vi "Passing Arrays as Read-Only ndarrays.vi"() -> ()   [LabVIEW 2020]
uses:
  6d5f1638-640c-4e20-b011-0cee3ae60b95.vi
  688a6956-cd2d-4b8a-a8be-e172edc5432f.vi
  G-Embedded-Python-Interpreter-Toolkit/Null Py Object Refnum.vi
  6d5f1638-640c-4e20-b011-0cee3ae60b95.vi/96ddca92-7bbf-40e2-a1a5-d32f291eb6af.vi
  688a6956-cd2d-4b8a-a8be-e172edc5432f.vi/6c7a13f1-33d3-431d-8188-904cac5422b3.vi
  G-Embedded-Python-Interpreter-Toolkit/Python Object Reference to Pointer Sized Ref.vi
  G-Embedded-Python-Interpreter-Toolkit/Pointer Sized Ref to Python Object Reference.vi
  G-Embedded-Python-Interpreter-Toolkit/Merge Call Library Errors.vi
  G-Embedded-Python-Interpreter-Toolkit/G-Embedded-Python-Interpreter-Toolkit.lvlib
panel:
  out "Average History":dbl(graph)
  out "Sample History":dbl[](graph)
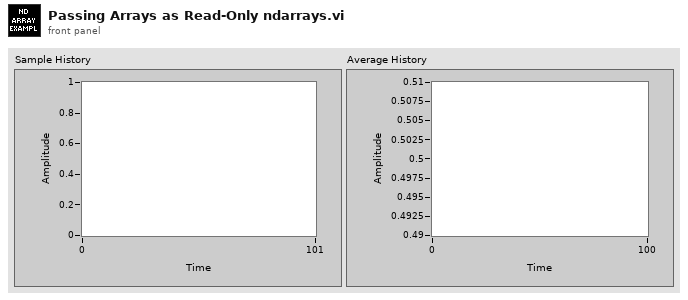
[diagram p1: front panel]
types:
  T1 = typedef "G-Embedded-Python-Interpreter-Toolkit.lvlib/Python Object Reference.ctl" = refnum<k1>
  T2 = typedef "G-Embedded-Python-Interpreter-Toolkit.lvlib/Type Information.ctl" = cluster{"Type":T3, "Array Dimensions":u8}
  T3 = typedef "NI_Data Type.lvlib/Data Type.ctl" = enum8{"Invalid Type", "Void", "I8", "I16", "I32", "I64", "U8", "U16", "U32", "U64", "Single Float", "Double Float", "Extended Float", "Single Complex", "Double Complex", "Extended Complex", "Enum U8", "Enum U16", "Enum U32", "Enum U64", "Single Float With Unit", "Double Float With Unit", "Extended Float With Unit", "Single Complex with Unit", "Double Complex with Unit", "Extended Complex with Unit", "Boolean", "String", "Path", "Picture", "Tag", "Array", "Cluster", "Variant", "LV Variant", "Waveform", "Timestamp", "Digital Waveform", "Digital Data", "ExpressData", "Refnum", "External Data", "VI", "Poly VI", "LabVIEW Class Instance", "Fixed Point", "Set Collection", "Map Collection"}
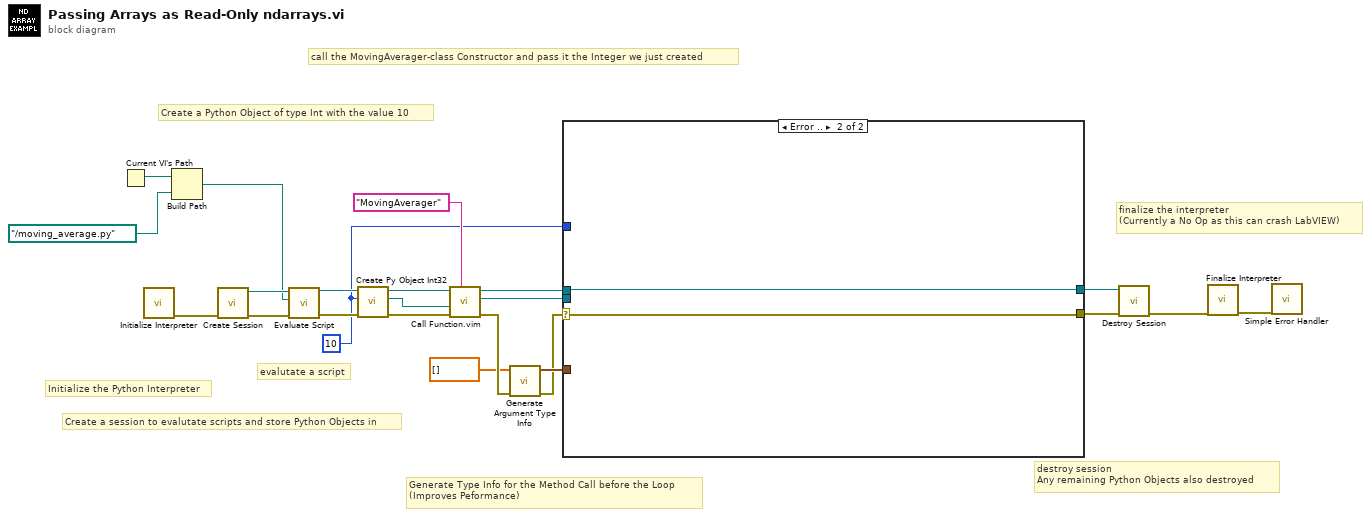
[diagram p0: block diagram]
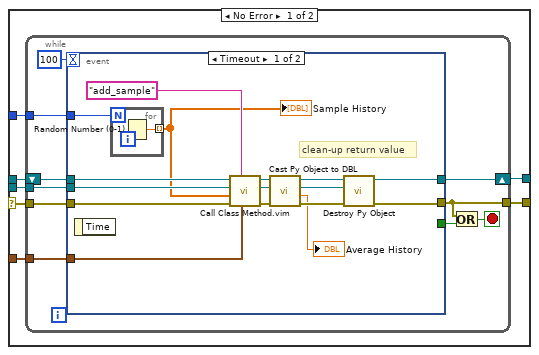
[diagram p2: hidden frame]
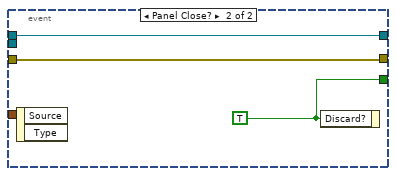
[diagram p3: hidden frame]
diagram:
  w12 = 10 ("Value")
  # "Generate Type Info for the Method Call before the Loop\n(Improves Peformance)"
  # "finalize the interpreter\n(Currently a No Op as this can crash LabVIEW)"
  # "destroy session \nAny remaining Python Objects also destroyed"
  # "Create a Python Object of type Int with the value 10"
  # "call the MovingAverager-class Constructor and pass it the Integer we just created"
  # "evalutate a script"
  # "Create a session to evalutate scripts and store Python Objects in"
  # "Initialize the Python Interpreter"
  n1 = Current VI's Path() -> (path=w20:path)
  n2 = call "Initialize Interpreter.vi"() -> ("error out"=w23:errorcluster)  [unwired: 10 in, 1 out]
  n3 = Build Path(base path=w20, name or relative path=path "../moving_average.py") -> (appended path=w18:path)
  n4 = call "Create Session.vi"("error in (no error)"=w23) -> ("error out"=w22:errorcluster, "Session Handle"=w21:refnum<data-value>)  [unwired: 9 in]
  n5 = call "Evaluate Script.vi"("error in (no error)"=w22, "Script File Path"=w18, "Session Handle in"=w21) -> ("error out"=w15:errorcluster, "Session Handle out"=w16:refnum<data-value>)  [unwired: 7 in]
  n6 = call "Create Py Object Int32.vi"("error in (no error)"=w15, "Value"=w12, "Session Handle in"=w16) -> ("error out"=w14:errorcluster, "Python Object Refnum"=w1:T1, "Session Handle out"=w13:refnum<data-value>)  [unwired: 6 in]
  n7 = call "Call Function.vim"("Function Name"="MovingAverager", "error in (no error)"=w14, "Arguments in (Default - None)"=w1, "Data Value Reference in"=w13) -> ("error out"=w4:errorcluster, "Returned Python Object Refnum"=w10:T1, "Data Value Reference out"=w11:refnum<data-value>)  [unwired: 5 in]
  n8 = call "Generate Argument Type Info.vi"("error in (no error)"=w4, "Data Type"=dbl[] []) -> ("error out"=w3:errorcluster, "Array"=w5:T2[])  [unwired: 8 in]
  n9 = case shown="Error .." w3 {
    selector: w3 -> [w30 w62]
    tunnel: w12 -> [w24 _]
    tunnel: w11 -> [w29 w61]
    tunnel: w10 -> [w28 _]
    tunnel: [w27 w62] -> w9
    tunnel: [w26 w61] -> w8
    tunnel: w5 -> [w25 _]
    frame No Error {
      n10 = while {
        tunnel: w30 -> [w40]
        shift-right: [w36] -> w26
        shift-left: w29 -> [w39]
        tunnel: w28 -> [w38]
        tunnel: [w34] -> w27
        tunnel: w25 -> [w33]
        tunnel: w24 -> [w32]
        stop <- w37 stop-if-true
        n11 = event shown="[0] Timeout" {
          selector: _ -> [_ _]
          dyn-events: _ -> [_ _]
          timeout: 100 -> [_ _]
          tunnel: w40 -> [w56 w60]
          tunnel: w39 -> [w55 w59]
          tunnel: w38 -> [w54 _]
          tunnel: [w46 w60] -> w34
          tunnel: [w45 w59] -> w36
          tunnel: [_ w58] -> w35
          tunnel: w33 -> [w44 _]
          tunnel: w32 -> [w43 _]
          event Timeout {
            # "clean-up return value"
            n12 = event-data() -> ()  [unwired: 1 in, 1 out]
            n13 = for {
              N: w43 -> [_]
              tunnel: [w57] -> w41 mode=indexing
              n14 = Random Number (0-1)() -> (number: 0 to 1=w57:dbl)
            }
            "Sample History" <- w41
            n15 = call "Call Class Method.vim"("Args Cluster Type Info (Empty - Generate)"=w44, "Function Name"="add_sample", "error in (no error)"=w56, "Arguments in (Default - Empty)"=w41, "Class Instance"=w54, "Data Value Reference in"=w55) -> ("error out"=w52:errorcluster, "Returned Python Object Refnum"=w50:T1, "Data Value Reference out"=w51:refnum<data-value>)  [unwired: 3 in]
            n16 = call "Cast Py Object to DBL.vi"("error in (no error)"=w52, "Python Object Refnum in"=w50, "Session Handle in"=w51) -> ("error out"=w47:errorcluster, "Value"=→"Average History":dbl, "Python Object Refnum out"=w48:T1, "Session Handle out"=w49:refnum<data-value>)  [unwired: 5 in]
            n17 = call "Destroy Py Object.vi"("error in (no error)"=w47, "Python Object Refnum"=w48, "Session Handle in"=w49) -> ("error out"=w46:errorcluster, "Session Handle out"=w45:refnum<data-value>)  [unwired: 7 in]
          }
          event Panel Close? {
            w58 = TRUE ("Discard?")
            n18 = event-data() -> ()  [unwired: 1 in, 2 out]
            n19 = event-data("Discard?"=w58) -> ()  [unwired: 1 in, 1 out]
          }
        }
        n20 = Or(x=w34, y=w35) -> (x .or. y?=w37:bool)
      }
    }
    frame Error {
    }
  }
  n21 = call "Destroy Session.vi"("error in (no error)"=w9, "Session Handle"=w8) -> ("error out"=w7:errorcluster)  [unwired: 9 in]
  n22 = call "Finalize Interpreter.vi"("error in (no error)"=w7) -> ("error out"=w6:errorcluster)  [unwired: 10 in]
  n23 = call <vilib>:"Simple Error Handler.vi"("error in (no error)"=w6) -> ()  [unwired: 4 in, 5 out]
